vi "Write (State).vi"(8 "error in (no error)":errorcluster, 10 "Value in":refnum<class "State.lvclass">, 11 "State in":refnum<class "State.lvclass">) -> (0 "error out":errorcluster, 2 "Value out":refnum<class "State.lvclass">, 3 "State out":refnum<class "State.lvclass">)   [LabVIEW 2017, in "Promise Future.lvlib" / "State.lvclass"]
uses:
  State.lvclass
  State.lvclass/State.ctl
  <vilib>/Utility/error.llb/Error Cluster From Error Code.vi
  <vilib>/ErrorRing/Error Ring.xnode
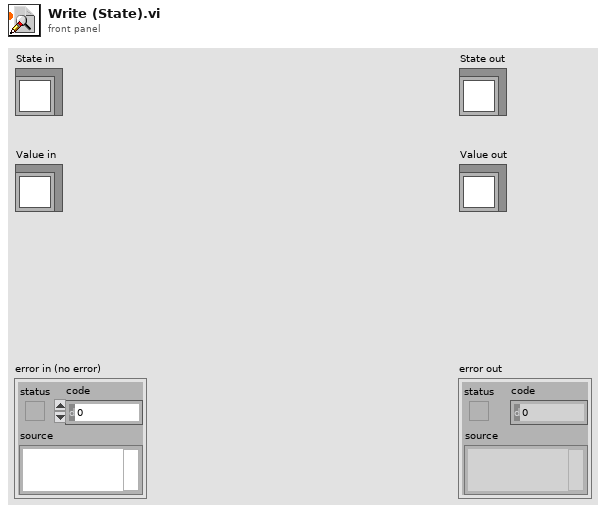
[diagram p1: front panel]
types:
  T1 = typedef "Promise.lvlib/State.lvclass/State Core.ctl" = cluster{"Value":refnum<queue>, "Callbacks":refnum<queue>, "Semaphore":T2}
  T2 = typedef "Semaphore RefNum" = refnum<k1>
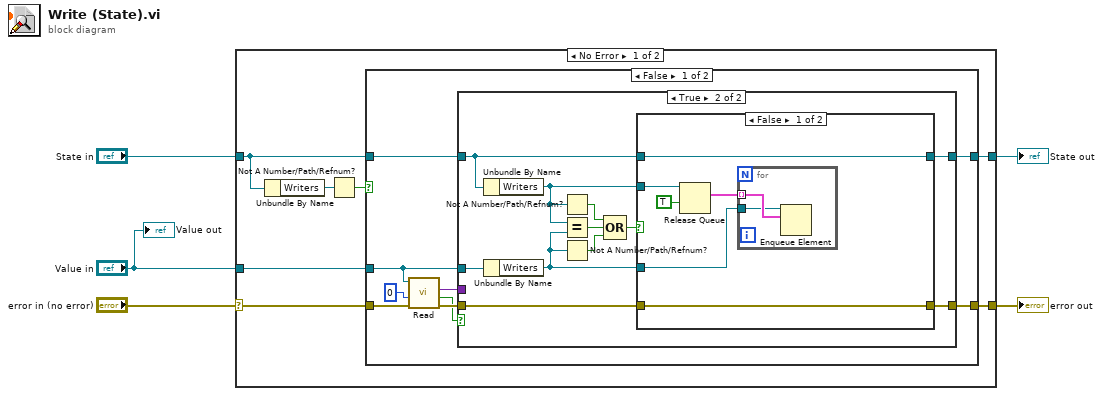
[diagram p0: block diagram]
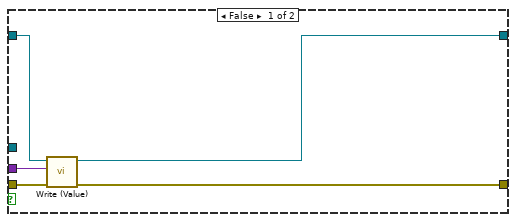
[diagram p2: hidden frame]
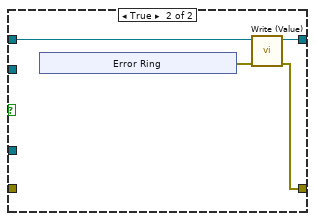
[diagram p3: hidden frame]
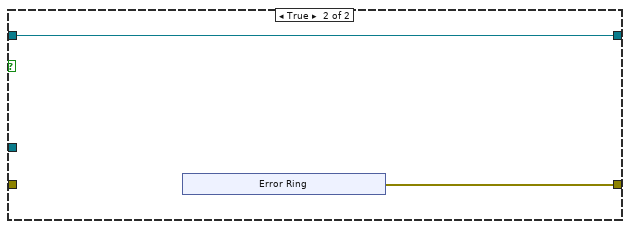
[diagram p4: hidden frame]
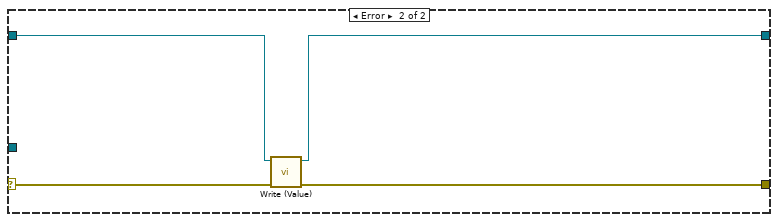
[diagram p5: hidden frame]
diagram:
  n1 = case shown="No Error" "error in (no error)" {
    selector: "error in (no error)" -> [w10 w65]
    tunnel: [w12 w63] -> w5
    tunnel: "State in" -> [w7 w62]
    tunnel: [w11 w64] -> w3
    tunnel: "Value in" -> [w9 _]
    frame No Error {
      n2 = Unbundle By Name(w7) -> ("Writers"=w8:refnum<queue>)
      n3 = Not A Number/Path/Refnum?(number/path/refnum=w8) -> (NaN/Path/Refnum?=w6:bool)
      n4 = case shown="False" w6 {
        tunnel: [w21 w56] -> w12
        tunnel: [w20 w55] -> w11
        tunnel: w9 -> [w18 _]
        tunnel: w7 -> [w19 w56]
        tunnel: w10 -> [w13 _]
        frame False {
          n5 = call "Read.vi"("error in (no error)"=w13, "timeout in ms (-1)"=0, "State in"=w18) -> ("error out"=w17:errorcluster, "timed out?"=w15:bool, "Value"=w14:variant)  [unwired: 6 in]
          n6 = case shown="True" w15 {
            tunnel: w19 -> [w26 w37]
            tunnel: [w25 w35] -> w21
            tunnel: w18 -> [_ w36]
            tunnel: w17 -> [w23 w29]
            tunnel: [w24 w30] -> w20
            tunnel: w14 -> [w22 _]
            frame False {
              n7 = call "Write (Value).vi"("error in (no error)"=w23, "Value"=w22, "State in"=w26) -> ("error out"=w24:errorcluster, "State out"=w25:refnum<class "State.lvclass">)  [unwired: 7 in]
            }
            frame True {
              n8 = Unbundle By Name(w37) -> ("Writers"=w31:refnum<queue>)
              n9 = Unbundle By Name(w36) -> ("Writers"=w34:refnum<queue>)
              n10 = Not A Number/Path/Refnum?(number/path/refnum=w31) -> (NaN/Path/Refnum?=w27:bool)
              n11 = Equal?(x=w31, y=w34) -> (x = y?=w33:bool)
              n12 = Not A Number/Path/Refnum?(number/path/refnum=w34) -> (NaN/Path/Refnum?=w28:bool)
              n13 = Compound Arithmetic op=OR(w27, w33, w28) -> (w32:bool)
              n14 = case shown="False" w32 {
                tunnel: w37 -> [w43 w49]
                tunnel: [w43 w48] -> w35
                tunnel: w34 -> [w42 _]
                tunnel: w31 -> [w41 _]
                tunnel: [w38 w46] -> w30
                tunnel: w29 -> [w38 _]
                frame False {
                  n15 = Release Queue(queue=w41, force destroy? (F)=TRUE) -> (remaining elements=w40:T1[])  [unwired: 1 in, 2 out]
                  n16 = for {
                    tunnel: w40 -> [w45] mode=indexing
                    tunnel: w42 -> [w44]
                    n17 = Enqueue Element(queue=w44, element=w45) -> ()  [unwired: 2 in, 3 out]
                  }
                }
                frame True {
                  n18 = xnode "Error Ring"() -> ("error out"=w47:errorcluster)
                  n19 = call "Write (Value).vi"("error in (no error)"=w47, "State in"=w49) -> ("error out"=w46:errorcluster, "State out"=w48:refnum<class "State.lvclass">)  [unwired: 8 in]
                }
              }
            }
          }
        }
        frame True {
          n20 = xnode "Error Ring"() -> ("error out"=w55:errorcluster)
        }
      }
    }
    frame Error {
      n21 = call "Write (Value).vi"("error in (no error)"=w65, "State in"=w62) -> ("error out"=w64:errorcluster, "State out"=w63:refnum<class "State.lvclass">)  [unwired: 8 in]
    }
  }
  "error out" <- w3
  "State out" <- w5
  "Value out" <- "Value in"
